vi "Check Escala.vi"(8 "error in (no error)":errorcluster, 10 "Grandeza":string, 11 "289 in":refnum<class "289.lvclass">) -> (0 "error out":errorcluster, 2 "Escala Correta?":bool, 3 "289 out":refnum<class "289.lvclass">)   [LabVIEW 2015, in "289.lvclass"]
uses:
  289.lvclass
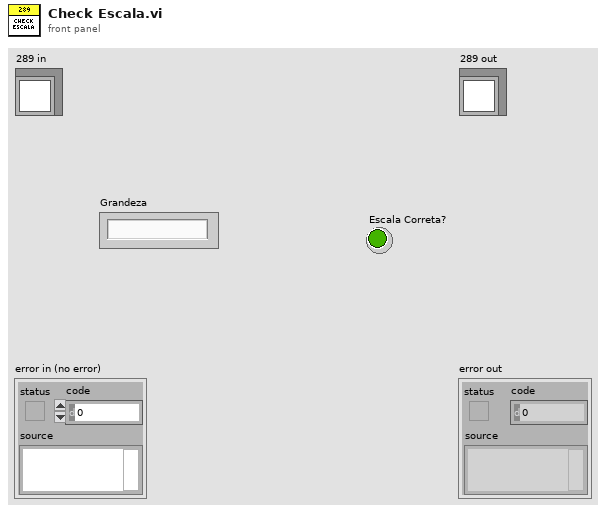
[diagram p1: front panel]
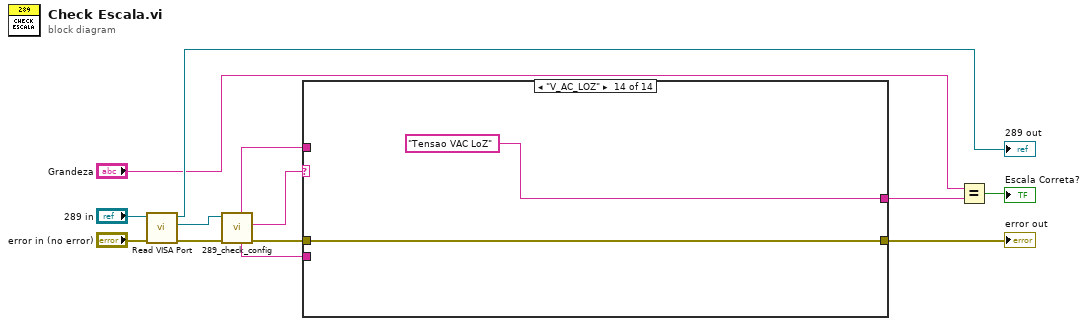
[diagram p0: block diagram]
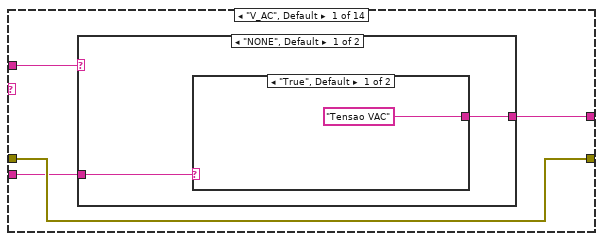
[diagram p2: hidden frame]
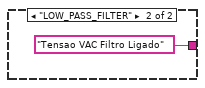
[diagram p3: hidden frame]
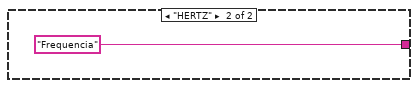
[diagram p4: hidden frame]
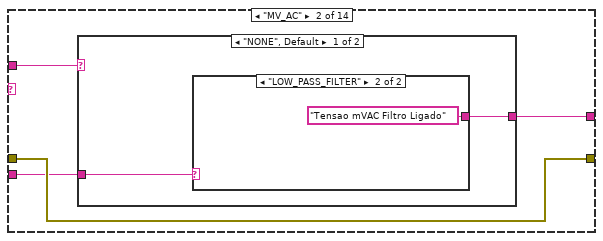
[diagram p5: hidden frame]
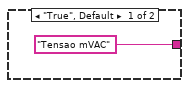
[diagram p6: hidden frame]
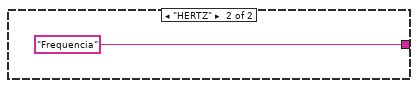
[diagram p7: hidden frame]
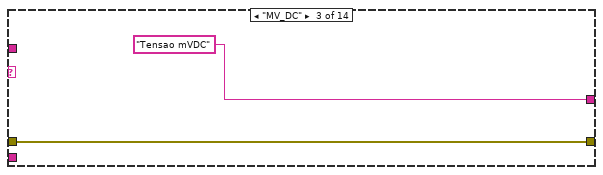
[diagram p8: hidden frame]
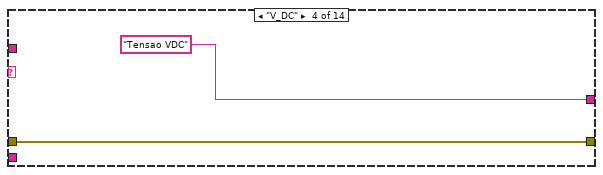
[diagram p9: hidden frame]
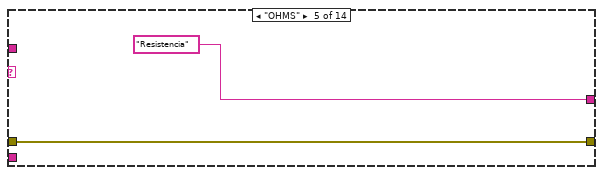
[diagram p10: hidden frame]
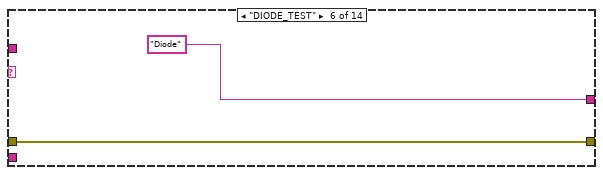
[diagram p11: hidden frame]
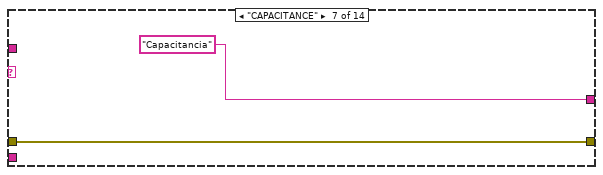
[diagram p12: hidden frame]
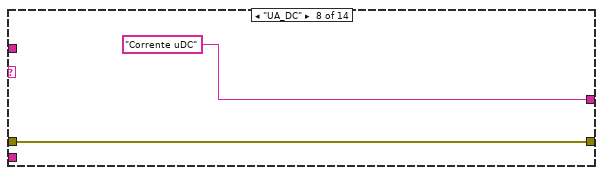
[diagram p13: hidden frame]
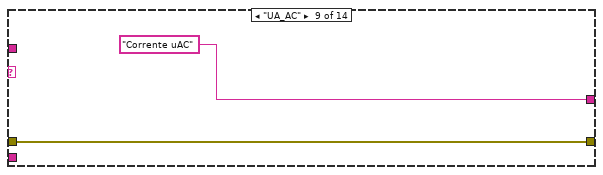
[diagram p14: hidden frame]
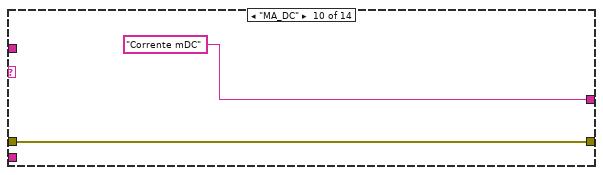
[diagram p15: hidden frame]
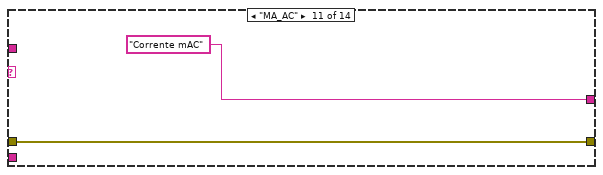
[diagram p16: hidden frame]
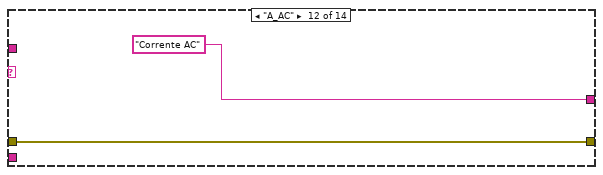
[diagram p17: hidden frame]
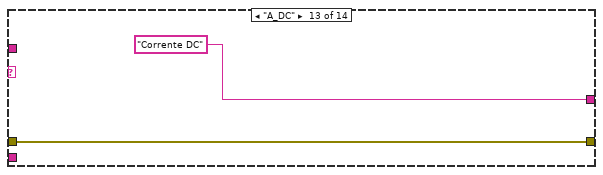
[diagram p18: hidden frame]
diagram:
  n1 = call-dynamic "Read VISA Port.vi"("error in (no error)"="error in (no error)", "Device in"="289 in") -> ("error out"=w11:errorcluster, "VISA Port"=w8:refnum<visa-resource-name>, "Device out"=→"289 out":refnum<class "289.lvclass">)  [unwired: 7 in]
  n2 = call "289_check_config.vi"("error in (no error)"=w11, "VISA resource name"=w8) -> ("error out"=w10:errorcluster, "Escala Principal"=w9:string, "Escala Secundária"=w1:string, "Secundária"=w2:string)  [unwired: 4 in, 2 out]
  n3 = case shown="\"V_AC_LOZ\"" w9 {
    tunnel: [w17 w26 w33 w35 w37 w39 w41 w43 w45 w47 w49 w51 w53 w55] -> w3
    tunnel: w10 -> [w17 w26 w33 w35 w37 w39 w41 w43 w45 w47 w49 w51 w53 w55]
    tunnel: [w16 w25 "Tensao mVDC" "Tensao VDC" "Resistencia" "Diode" "Capacitancia" "Corrente uDC" "Corrente uAC" "Corrente mDC" "Corrente mAC" "Corrente AC" "Corrente DC" "Tensao VAC LoZ"] -> w4
    tunnel: w2 -> [w15 w24 _ _ _ _ _ _ _ _ _ _ _ _]
    tunnel: w1 -> [w14 w23 _ _ _ _ _ _ _ _ _ _ _ _]
    frame "V_AC", Default {
      n4 = case shown="\"NONE\", Default" w15 {
        tunnel: [w19 "Frequencia"] -> w16
        tunnel: w14 -> [w18 _]
        frame "NONE", Default {
          n5 = case shown="\"True\", Default" w18 {
            tunnel: ["Tensao VAC" "Tensao VAC Filtro Ligado"] -> w19
            frame "True", Default {
            }
            frame "LOW_PASS_FILTER" {
            }
          }
        }
        frame "HERTZ" {
        }
      }
    }
    frame "MV_AC" {
      n6 = case shown="\"NONE\", Default" w24 {
        tunnel: [w28 "Frequencia"] -> w25
        tunnel: w23 -> [w27 _]
        frame "NONE", Default {
          n7 = case shown="\"LOW_PASS_FILTER\"" w27 {
            tunnel: ["Tensao mVAC" "Tensao mVAC Filtro Ligado"] -> w28
            frame "True", Default {
            }
            frame "LOW_PASS_FILTER" {
            }
          }
        }
        frame "HERTZ" {
        }
      }
    }
    frame "MV_DC" {
    }
    frame "V_DC" {
    }
    frame "OHMS" {
    }
    frame "DIODE_TEST" {
    }
    frame "CAPACITANCE" {
    }
    frame "UA_DC" {
    }
    frame "UA_AC" {
    }
    frame "MA_DC" {
    }
    frame "MA_AC" {
    }
    frame "A_AC" {
    }
    frame "A_DC" {
    }
    frame "V_AC_LOZ" {
    }
  }
  "error out" <- w3
  n8 = Equal?(x="Grandeza", y=w4) -> (x = y?=→"Escala Correta?":bool)
